vi "EPTxRTmul-inj3.vi"(3 "Cmd_Input":T1={"Cmd_Duration"={"Duration1"=2.0, "Duratiion2"=4.0, "Duration3"=2.0, "Duration4"=4.0, "Duration5"=16.0, "Duration6"=4.0, "Duration7"=2.0, "Duration8"=2.0}, "Cmd_Bool"={"Bool1"=TRUE, "Bool2"=TRUE, "Bool3"=TRUE}, "Speed (RPM)"=0.0} caption="簇") -> (1 "Cmd_Seq":T2)   [LabVIEW 2020]
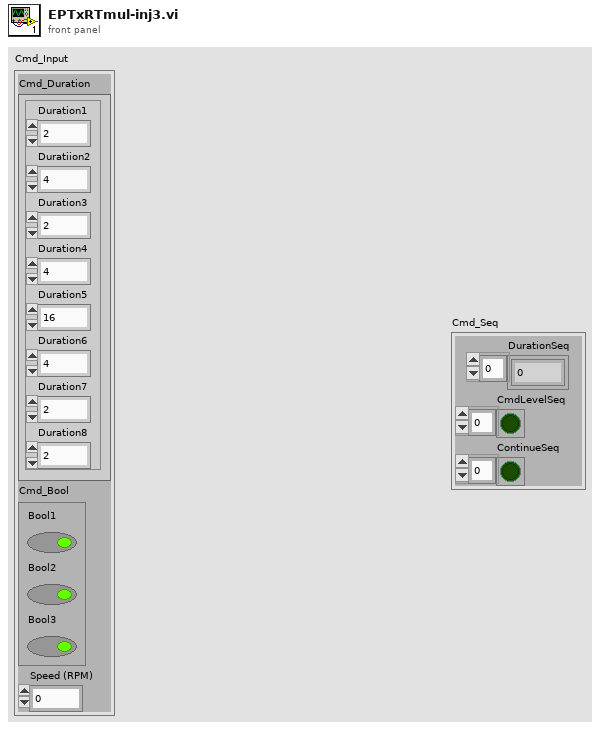
[diagram p1: front panel]
types:
  T1 = cluster{"Cmd_Duration":cluster{"Duration1":sgl, "Duratiion2":sgl, "Duration3":sgl, "Duration4":sgl, "Duration5":sgl, "Duration6":sgl, "Duration7":sgl, "Duration8":sgl}, "Cmd_Bool":cluster{"Bool1":bool, "Bool2":bool, "Bool3":bool}, "Speed (RPM)":sgl}
  T2 = cluster{"DurationSeq":u32[], "CmdLevelSeq":bool[], "ContinueSeq":bool[]}
  T3 = cluster{"Duration1":sgl, "Duratiion2":sgl, "Duration3":sgl, "Duration4":sgl, "Duration5":sgl, "Duration6":sgl, "Duration7":sgl, "Duration8":sgl}
  T4 = cluster{"Bool1":bool, "Bool2":bool, "Bool3":bool}
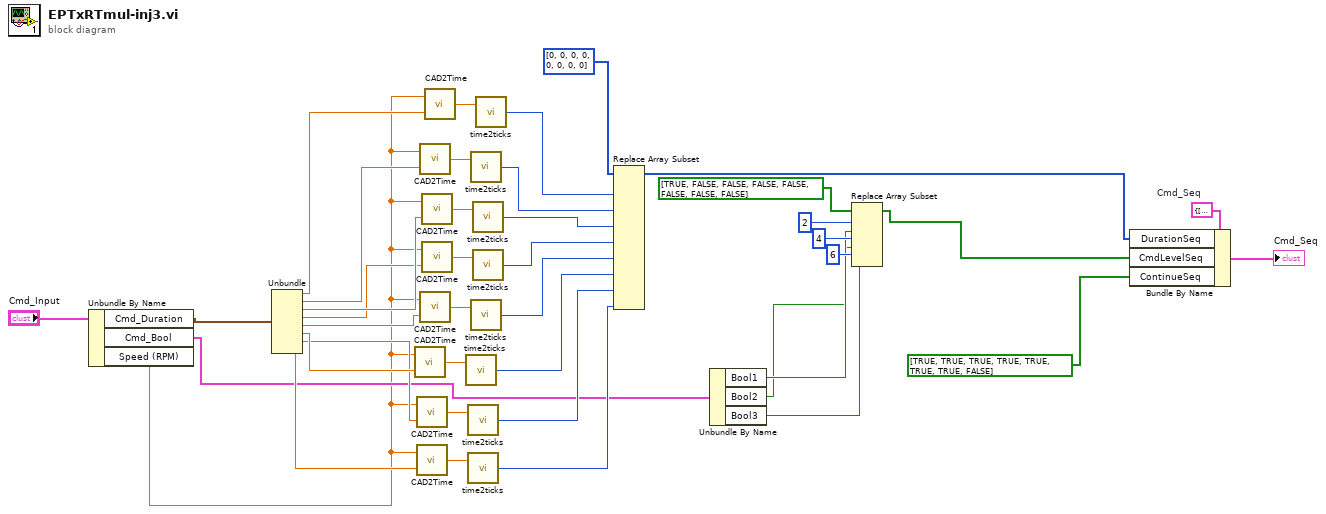
[diagram p0: block diagram]
diagram:
  w36 = T2 {"DurationSeq"=[0, 0, 0, 0, 0, 0, 0, 0], "CmdLevelSeq"=[FALSE, FALSE, FALSE, FALSE, FALSE, FALSE, FALSE, FALSE], "ContinueSeq"=[FALSE, FALSE, FALSE, FALSE, FALSE, FALSE, FALSE, FALSE]}  # Cmd_Seq
  n1 = Unbundle By Name("Cmd_Input") -> ("Cmd_Duration"=w3:T3, "Cmd_Bool"=w2:T4, "Speed (RPM)"=w1:sgl)
  n2 = Unbundle(w3) -> ("Duration1"=w32:sgl, "Duratiion2"=w25:sgl, "Duration3"=w24:sgl, "Duration4"=w23:sgl, "Duration5"=w22:sgl, "Duration6"=w21:sgl, "Duration7"=w20:sgl, "Duration8"=w19:sgl)
  n3 = call <vilib>:"CAD2Time.vi"("CAD"=w21, "Speed (RPM)"=w1) -> ("Time [ms]"=w27:sgl)
  n4 = call <vilib>:"CAD2Time.vi"("CAD"=w20, "Speed (RPM)"=w1) -> ("Time [ms]"=w28:sgl)
  n5 = call <vilib>:"CAD2Time.vi"("CAD"=w19, "Speed (RPM)"=w1) -> ("Time [ms]"=w29:sgl)
  n6 = call <vilib>:"CAD2Time.vi"("CAD"=w25, "Speed (RPM)"=w1) -> ("Time [ms]"=w33:sgl)
  n7 = call <vilib>:"CAD2Time.vi"("CAD"=w22, "Speed (RPM)"=w1) -> ("Time [ms]"=w26:sgl)
  n8 = call <vilib>:"CAD2Time.vi"("CAD"=w24, "Speed (RPM)"=w1) -> ("Time [ms]"=w31:sgl)
  n9 = call <vilib>:"CAD2Time.vi"("CAD"=w23, "Speed (RPM)"=w1) -> ("Time [ms]"=w30:sgl)
  n10 = call <vilib>:"CAD2Time.vi"("CAD"=w32, "Speed (RPM)"=w1) -> ("Time [ms]"=w37:sgl)
  n11 = call <vilib>:"time2ticks.vi"("Time (msec)"=w27) -> ("Ticks"=w11:u32)  [unwired: 1 in]
  n12 = call <vilib>:"time2ticks.vi"("Time (msec)"=w28) -> ("Ticks"=w10:u32)  [unwired: 1 in]
  n13 = call <vilib>:"time2ticks.vi"("Time (msec)"=w29) -> ("Ticks"=w9:u32)  [unwired: 1 in]
  n14 = call <vilib>:"time2ticks.vi"("Time (msec)"=w33) -> ("Ticks"=w15:u32)  [unwired: 1 in]
  n15 = call <vilib>:"time2ticks.vi"("Time (msec)"=w26) -> ("Ticks"=w12:u32)  [unwired: 1 in]
  n16 = call <vilib>:"time2ticks.vi"("Time (msec)"=w31) -> ("Ticks"=w14:u32)  [unwired: 1 in]
  n17 = call <vilib>:"time2ticks.vi"("Time (msec)"=w30) -> ("Ticks"=w13:u32)  [unwired: 1 in]
  n18 = call <vilib>:"time2ticks.vi"("Time (msec)"=w37) -> ("Ticks"=w16:u32)  [unwired: 1 in]
  n19 = Replace Array Subset(array=u32[] [0, 0, 0, 0, 0, 0, 0, 0] ("DurationSeq"), new element #1=w16, new element #2=w15, new element #3=w14, new element #4=w13, new element #5=w12, new element #6=w11, new element #7=w10, new element #8=w9) -> (w17:u32[])  [unwired: 8 in]
  n20 = Unbundle By Name(w2) -> ("Bool1"=w8:bool, "Bool2"=w7:bool, "Bool3"=w6:bool)
  n21 = Replace Array Subset ("替换数组子集")(array=bool[] [TRUE, FALSE, FALSE, FALSE, FALSE, FALSE, FALSE, FALSE] ("CmdLevel"), new element #1=w8, index #1=2 ("index"), new element #2=w7, index #2=4 ("index"), new element #3=w6, index #3=6 ("index")) -> (w35:bool[])
  n22 = Bundle By Name(cluster=w36, "DurationSeq"=w17, "CmdLevelSeq"=w35, "ContinueSeq"=bool[] [TRUE, TRUE, TRUE, TRUE, TRUE, TRUE, TRUE, FALSE] ("Continue")) -> (→"Cmd_Seq":T2)
